vi "Corner Detection.vi"() -> ()   [LabVIEW 2018]
doc: "Corner Detection: This example is a corner detection example used to locate and recognize corners (also known as points of interest) in images or image sequences. Corner points usually refer to the positions in an image where significant changes occur within a local area."
uses:
  vi.lib/VIRobotics/opencv_yiku/ctls/ColorConversionCodes.ctl
  vi.lib/VIRobotics/opencv_yiku/Mat/Create_Mat_8U.vi
  vi.lib/VIRobotics/opencv_yiku/Mat/Mat_8U/set2ddata.vi
  vi.lib/VIRobotics/opencv_yiku/Mat/Mat_8U/Mat_8U.lvclass
  vi.lib/VIRobotics/opencv_yiku/opencv_yiku.lvlib
panel:
  out "picture":picture
  out "corner":picture
  out "max value":sgl
  out "dst":sgl[][](array[numeric])
  # "Overview: Demonstrates how to finish Corner Detection\nRequirements: Windows.\nInstructions: \n1.Run the VI"
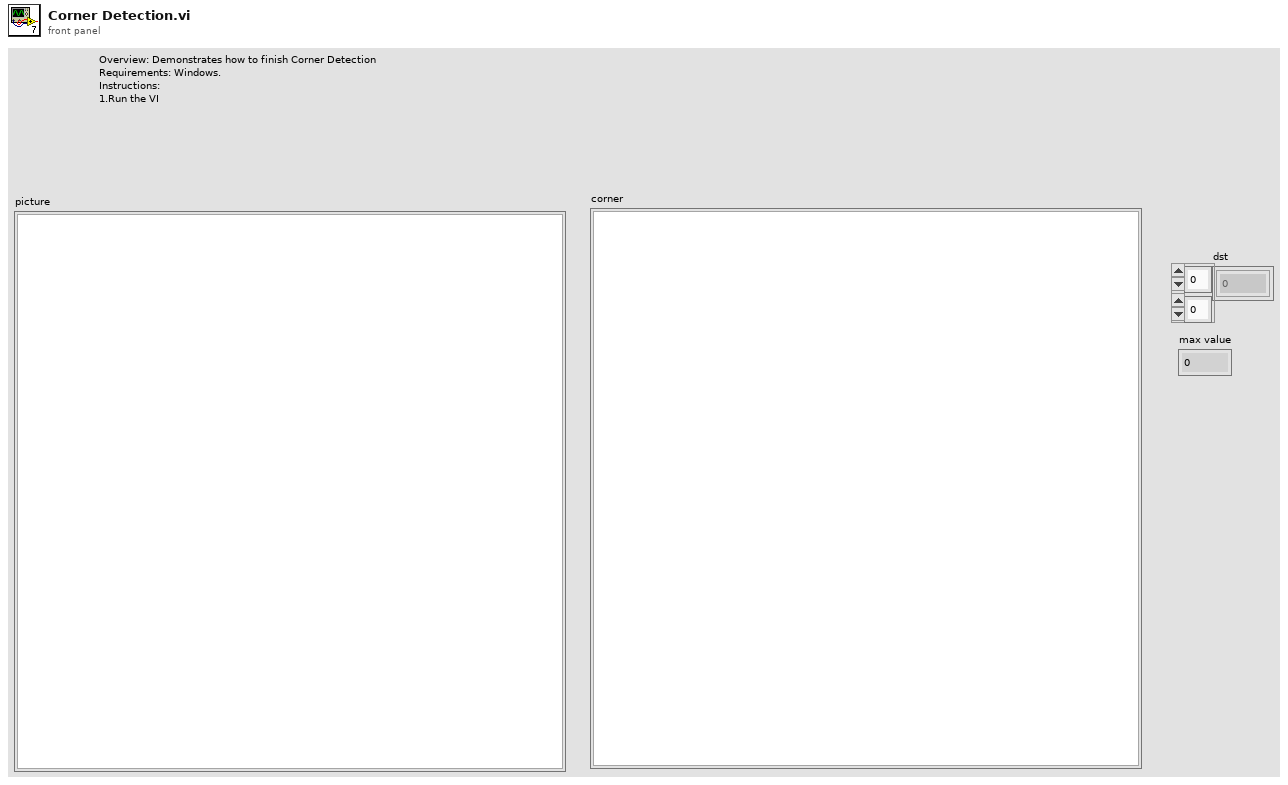
[diagram p1: front panel]
types:
  T1 = typedef "opencv_yiku.lvlib/ColorConversionCodes.ctl" = enum32{"COLOR_BGR2BGRA", "COLOR_BGRA2BGR", "COLOR_BGR2RGBA", "COLOR_RGBA2BGR", "COLOR_BGR2RGB", "COLOR_BGRA2RGBA", "COLOR_BGR2GRAY", "COLOR_RGB2GRAY", "COLOR_GRAY2BGR", "COLOR_GRAY2BGRA", "COLOR_BGRA2GRAY", "COLOR_RGBA2GRAY", "COLOR_BGR2BGR565", "COLOR_RGB2BGR565", "COLOR_BGR5652BGR", "COLOR_BGR5652RGB", "COLOR_BGRA2BGR565", "COLOR_RGBA2BGR565", "COLOR_BGR5652BGRA", "COLOR_BGR5652RGBA", "COLOR_GRAY2BGR565", "COLOR_BGR5652GRAY", "COLOR_BGR2BGR555", "COLOR_RGB2BGR555", "COLOR_BGR5552BGR", "COLOR_BGR5552RGB", "COLOR_BGRA2BGR555", "COLOR_RGBA2BGR555", "COLOR_BGR5552BGRA", "COLOR_BGR5552RGBA", "COLOR_GRAY2BGR555", "COLOR_BGR5552GRAY", "COLOR_BGR2XYZ", "COLOR_RGB2XYZ", "COLOR_XYZ2BGR", "COLOR_XYZ2RGB", "COLOR_BGR2YCrCb", "COLOR_RGB2YCrCb", "COLOR_YCrCb2BGR", "COLOR_YCrCb2RGB", "COLOR_BGR2HSV", "COLOR_RGB2HSV", "42", "43", "COLOR_BGR2Lab", "COLOR_RGB2Lab"}
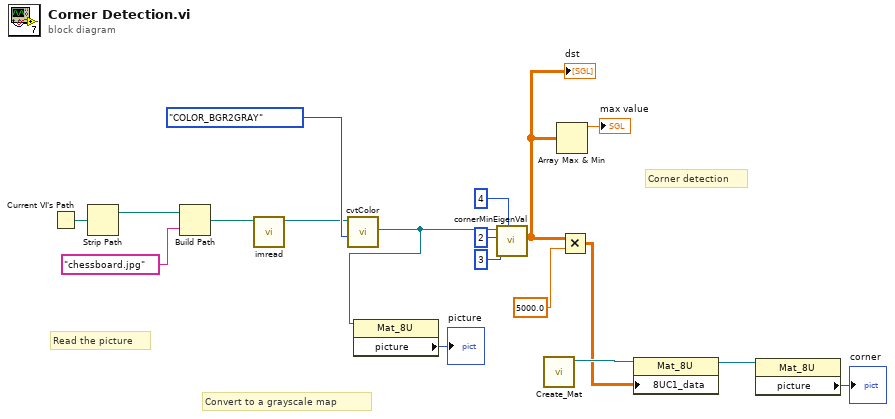
[diagram p0: block diagram]
diagram:
  # "Corner detection"
  # "Convert to a grayscale map"
  # "Read the picture"
  n1 = Current VI's Path() -> (path=w17:path)
  n2 = Strip Path(path=w17) -> (stripped path=w18:path)  [unwired: 1 out]
  n3 = Build Path(base path=w18, name or relative path="chessboard.jpg") -> (appended path=w15:path)
  n4 = call "imread.vi"("path"=w15) -> ("Mat out"=w2:refnum<class "Mat_8U.lvclass">)  [unwired: 9 in, 1 out]
  n5 = call "cvtColor.vi"("dstCn"=ColorConversionCodes."COLOR_BGR2GRAY", "src"=w2) -> ("dst out"=w1:refnum<class "Mat_8U.lvclass">)  [unwired: 7 in, 2 out]
  n6 = property class="Mat_8U"(reference=w1) -> ("picture"=→"picture":picture)  [unwired: 1 in, 2 out]
  n7 = call "cornerMinEigenVal.vi"("borderType"=4, "ksize"=3, "blocksize"=2, "src"=w1) -> ("dst"=w8:sgl[][])  [unwired: 5 in, 2 out]
  "dst" <- w8
  n8 = call-poly "Create_Mat.vi"() -> ("Mat_8U_out"=w7:refnum<class "Mat_8U.lvclass">)  [unwired: 10 in, 1 out]
  n9 = Array Max & Min(array=w8) -> (max value=→"max value":sgl)  [unwired: 3 out]
  n10 = Multiply(x=w8, y=sgl 5000.0) -> (x*y=w6:sgl[][])
  n11 = property class="Mat_8U"(reference=w7, "8UC1_data"=w6) -> (reference out=w5:refnum<class "Mat_8U.lvclass">)  [unwired: 1 in, 1 out]
  n12 = property class="Mat_8U"(reference=w5) -> ("picture"=→"corner":picture)  [unwired: 1 in, 2 out]
